vi "ShiftOrigin.vi"(0 "reference in":refnum<class "LcPictureBox.lvclass">, 2 "Delta(raw)":cluster{"x":sgl, "y":sgl}, 5 "Error In":errorcluster) -> (14 "reference out":refnum<class "LcPictureBox.lvclass">, 16 "Origin":cluster{"x":sgl, "y":sgl}, 19 "Error Out":errorcluster)   [LabVIEW 2020, in "LcPictureBox.lvclass"]
uses:
  LcPictureBox.lvclass
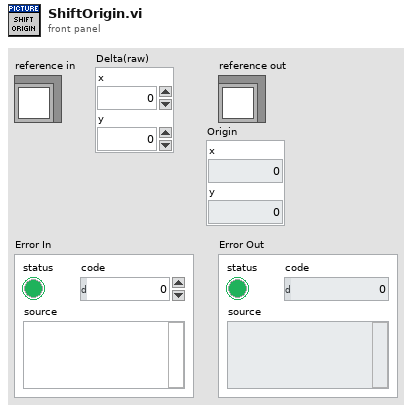
[diagram p1: front panel]
types:
  T1 = typedef "LcPictureBox.lvclass/ObjectAttributes.ctl" = cluster{"PictureBox":refnum<k24>, "ImageSize":cluster{"Width":i32, "Height":i32}, "PenMemory":map{cluster{"Alpha(100%)":dbl, "Color(Black)":u32, "Pen(Width=1, Solid)":T2}, refnum<k24>}, "GraphicsRef":refnum<k24>, "BrushMemory":map{cluster{"Alpha(100%)":dbl, "Color(Black)":u32}, refnum<k24>}, "Images":refnum<k24>[], "ImageIndex":i32, "BgColor(None)":u32, "LoadedImages":map{string, cluster{"ImageOut":refnum<k24>, "ImageSize":cluster{"Width":i32, "Height":i32}}}, "ColorsMemory":map{cluster{"Alpha(100%)":dbl, "Color(Black)":u32}, refnum<k24>}, "CacheSize":i32, "PictureBoxActiveXReference":refnum<vi>, "Scale":sgl, "Offset":cluster{"x":sgl, "y":sgl}, "zoom_center":cluster{"X":i32, "Y":i32}, "ImagesCreated":refnum<k24>[]}
  T2 = typedef "LcPictureBox.lvclass/Pen.ctl" = cluster{"Width":u16, "Style":enum32{"Solid", "Dash", "Dot", "DashDot", "DashDotDot"}}
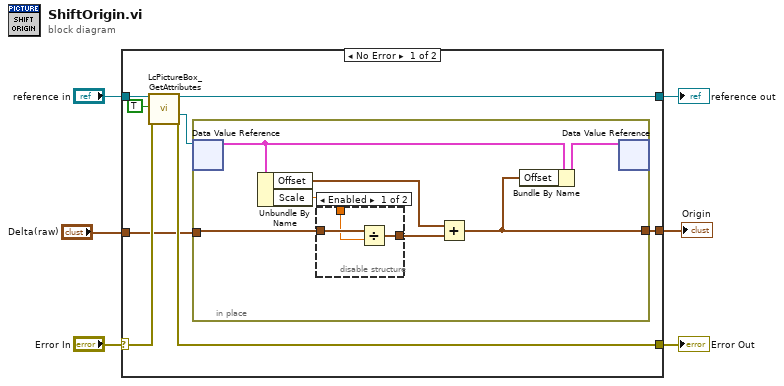
[diagram p0: block diagram]
diagram:
  n1 = case shown="No Error" "Error In" {
    selector: "Error In" -> [w14 w27]
    tunnel: [w13 w27] -> w5
    tunnel: [w11 w26] -> w3
    tunnel: "reference in" -> [w12 w26]
    tunnel: "Delta(raw)" -> [w8 _]
    tunnel: [w7 _] -> w1
    frame No Error {
      n2 = call "LcPictureBox_GetAttributes.vi"("reference in"=w12, "OnlyGetDvrReference(False)"=TRUE, "error in (no error)"=w14) -> ("reference out"=w11:refnum<class "LcPictureBox.lvclass">, "DataRef"=w10:refnum<data-value>, "error out"=w13:errorcluster)  [unwired: 13 in, 1 out]
      n3 = in-place {
        in-place-border: w8 -> [w18]
        in-place-border: [w15] -> w7
        n4 = in-place-dvr #1(w10) -> (w20:T1)  [unwired: 1 out]
        n5 = Unbundle By Name(w20) -> ("Offset"=w19:cluster{"x":sgl, "y":sgl}, "Scale"=w17:sgl)
        n6 = disable-structure shown="Enabled" {
          disable-tunnel: w18 -> [w24 w25]
          disable-tunnel: w17 -> [w23 _]
          disable-tunnel: [w22 w25] -> w16
          frame Enabled {
            n7 = Divide(x=w24, y=w23) -> (x/y=w22:cluster{"x":sgl, "y":sgl})
          }
          frame Disabled {
          }
        }
        n8 = Add(x=w19, y=w16) -> (x+y=w15:cluster{"x":sgl, "y":sgl})
        n9 = Bundle By Name(cluster=w20, "Offset"=w15) -> (w21:T1)
        n10 = in-place-dvr #1(w21) -> ()  [unwired: 2 out]
      }
    }
    frame Error {
    }
  }
  "Error Out" <- w5
  "reference out" <- w3
  "Origin" <- w1
